vi "Is Private Data Empty.vi"(8 "error in":errorcluster, 10 "Ref.Private Data Cluster":refnum<vi>) -> (0 "error out":errorcluster, 2 "Private Data Empty?":bool)   [LabVIEW 2021, in "_Msg Rescript.lvlib" / "_Msg Rescript.lvclass"]
uses:
  _Msg Rescript.lvclass
  _Msg Rescript.lvclass/_Msg Rescript.ctl
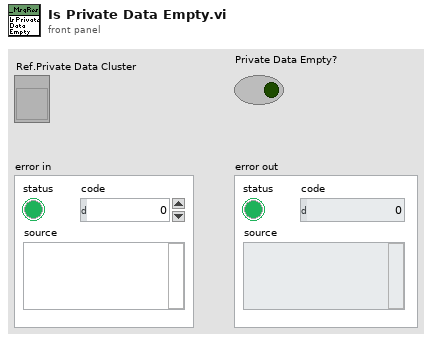
[diagram p1: front panel]
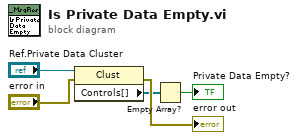
[diagram p0: block diagram]
diagram:
  n1 = property class="Clust"(reference="Ref.Private Data Cluster", error in="error in") -> (error out=→"error out":errorcluster, "Controls[]"=w2:refnum<vi>[])  [unwired: 1 out]
  n2 = Empty Array?(array=w2) -> (empty?=→"Private Data Empty?":bool)
